vi "Start_Stop Acq.vi"(6 "Start/Stop":enum16{"Start", "Stop"}(ring), 8 "error in":errorcluster, 11 "4300 in":refnum<class "4300.lvclass">) -> (0 "error out":errorcluster, 3 "4300 out":refnum<class "4300.lvclass">)   [LabVIEW 2019, in "4300.lvlib" / "4300.lvclass"]
doc: "Implements start stop acquisition functionality of PXIe 4300"
uses:
  Library/4300.lvclass
  Library/4300.lvclass/4300.ctl
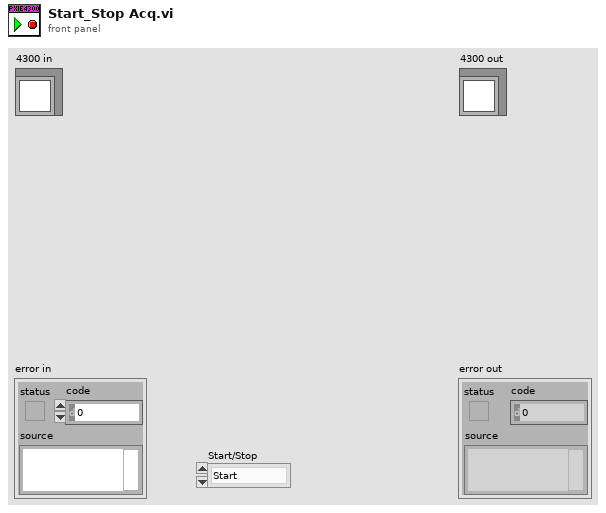
[diagram p1: front panel]
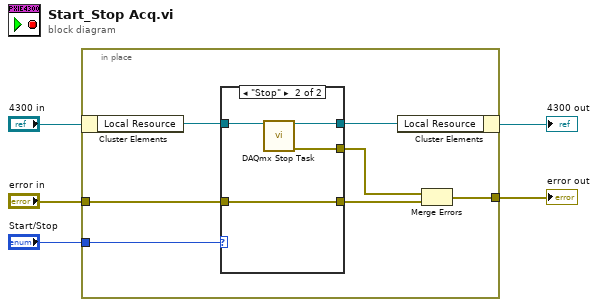
[diagram p0: block diagram]
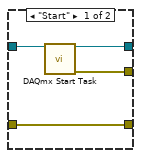
[diagram p2: hidden frame]
diagram:
  n1 = in-place {
    in-place-border: "error in" -> [w7]
    in-place-border: "Start/Stop" -> [w12]
    in-place-border: [w8] -> w1
    n2 = in-place-cluster #1("4300 in") -> ("Local Resource"=w11:refnum<k21>)
    n3 = case shown="\"Stop\"" w12 {
      tunnel: [w15 w19] -> w10
      tunnel: w11 -> [w16 w20]
      tunnel: [w14 w18] -> w9
      tunnel: w7 -> [w13 w17]
      tunnel: [w13 w17] -> w6
      frame "Start" {
        # "Start Data Acquisition."
        n4 = call <vilib>:"DAQmx Start Task.vi"("task/channels in"=w16) -> ("task out"=w15:refnum<k21>, "error out"=w14:errorcluster)  [unwired: 13 in]
      }
      frame "Stop" {
        # "Stop acquisition even if there is an error on the incoming terminal"
        n5 = call <vilib>:"DAQmx Stop Task.vi"("task/channels in"=w20) -> ("task out"=w19:refnum<k21>, "error out"=w18:errorcluster)  [unwired: 13 in]
      }
    }
    n6 = in-place-cluster #1("Local Resource"=w10) -> (→"4300 out":refnum<class "4300.lvclass">)
    n7 = Merge Errors(w9, w6) -> (w8:errorcluster)
  }
  "error out" <- w1
